vi "mac EXT ARMS TO MISS INTAKE.vi"(8 "error in (no error)":errorcluster) -> (0 "error out":errorcluster)   [LabVIEW 2020]
doc: "macro to climb from the ground to the MID bar"
uses:
  ctrl ARM MACRO ENTRY.ctl
  Robot Global Data.vi
panel:
  out "dist to extend above clearance (in)":dbl[](array[numeric])=[17.112499999999997, 13.487499999999997]
  out "clearance ht req'd (in AG)":dbl=62.125
  out "HANGAR BARS":T1={"LOW BAR AG"=48.75, "MID BAR AG"=60.25, "HIGH BAR AG"=75.625, "TRAV BAR AG"=91.0, "BAR OD"=1.66, "SPACING"=24.0}
  out "ARM Climber range":T2={"MIN"=0.0, "MAX"=22.5, "convert climber inches to tics"=18192.520379, "INITIALIZE"=-0.0625} {"convert climber inches to tics" format="%.6g"}
  out "ARM angle range":T3={"MIN"=-3.5, "MAX"=4.5, "convert arm inches to revs"=42.857, "convert arm inches to degrees"=4.96493} {"convert arm inches to degrees" format="%.6g"; "convert arm inches to revs" format="%.6g"}
  out "ARM DIMS":T4={"HOOK CTR LENGTH LEFT"=38.1375, "HOOK CTR LENGTH RIGHT"=41.7625, "HOOK DEPTH"=2.0, "HOOK ID"=1.875, "SHOULDER PIN AG"=6.875, "ARM DIFF RT-LEFT"=3.625}
  in  "Array":T6(array[cluster])=[{"LEFT"={"Climber"={"skip?"=FALSE, "CLIMBER STROKE (in)"=2.0, " speed"=0.75}, "Angle"={"skip?"=TRUE, "ARM ANGLE (deg)"=0.0, " speed"=1.0}, "DELAY (ms)"=0}, "RIGHT"={"Climber"={"skip?"=FALSE, "CLIMBER STROKE (in)"=2.0, " speed"=0.75}, "Angle"={"skip?"=TRUE, "ARM ANGLE (deg)"=0.0, " speed"=1.0}, "DELAY (ms)"=0}, "comment"={"movement"="RAISE 2.0 INCHES", "descr"=""}}] {"RIGHT"."Angle"."speed" min=0.0 max=1.0 format="%_3g"; "RIGHT"."Angle"."ARM ANGLE (deg)" format="%.3g"; "RIGHT"."Climber"."CLIMBER STROKE (in)" format="%_5g"; "RIGHT"."Climber"."speed" min=0.0 max=1.0 format="%_3g"; "LEFT"."Angle"."speed" min=0.0 max=1.0 format="%_3g"; "LEFT"."Angle"."ARM ANGLE (deg)" format="%.3g"; "LEFT"."Climber"."CLIMBER STROKE (in)" format="%_5g"; "LEFT"."Climber"."speed" min=0.0 max=1.0 format="%_3g"}
  # "22-03-15  LOW HOOKS ID measured to be about 35.5\" above shoulder pin\n35.5 + 6.875 = 42.375\" AG\n48.75\" bar - 42.375\" top ID + 2\"D + 1\" clear = 9.375\""
  # "mac EXT ARMS for MID\nExtend & angle arms to climb the MID bar\n\n1) extend arms enough to clear MID bar and angle forward\n2) angle arms rearward\n3) retract arms 4\" to grab bar\n4) retract arms and angle back to 0; leave 0.375\" buffer on right arm\n\nDO NOT FORGET TO \"MAKE CURRENT VALUES DEFAULT\""
  # "22-03-14 measured arm lengths:\nat 0% stroke, the inside hook openings were\nLEFT = 40.375\"  and RIGHT = 44.0\"\nwrt top of the shoulder arm plate"
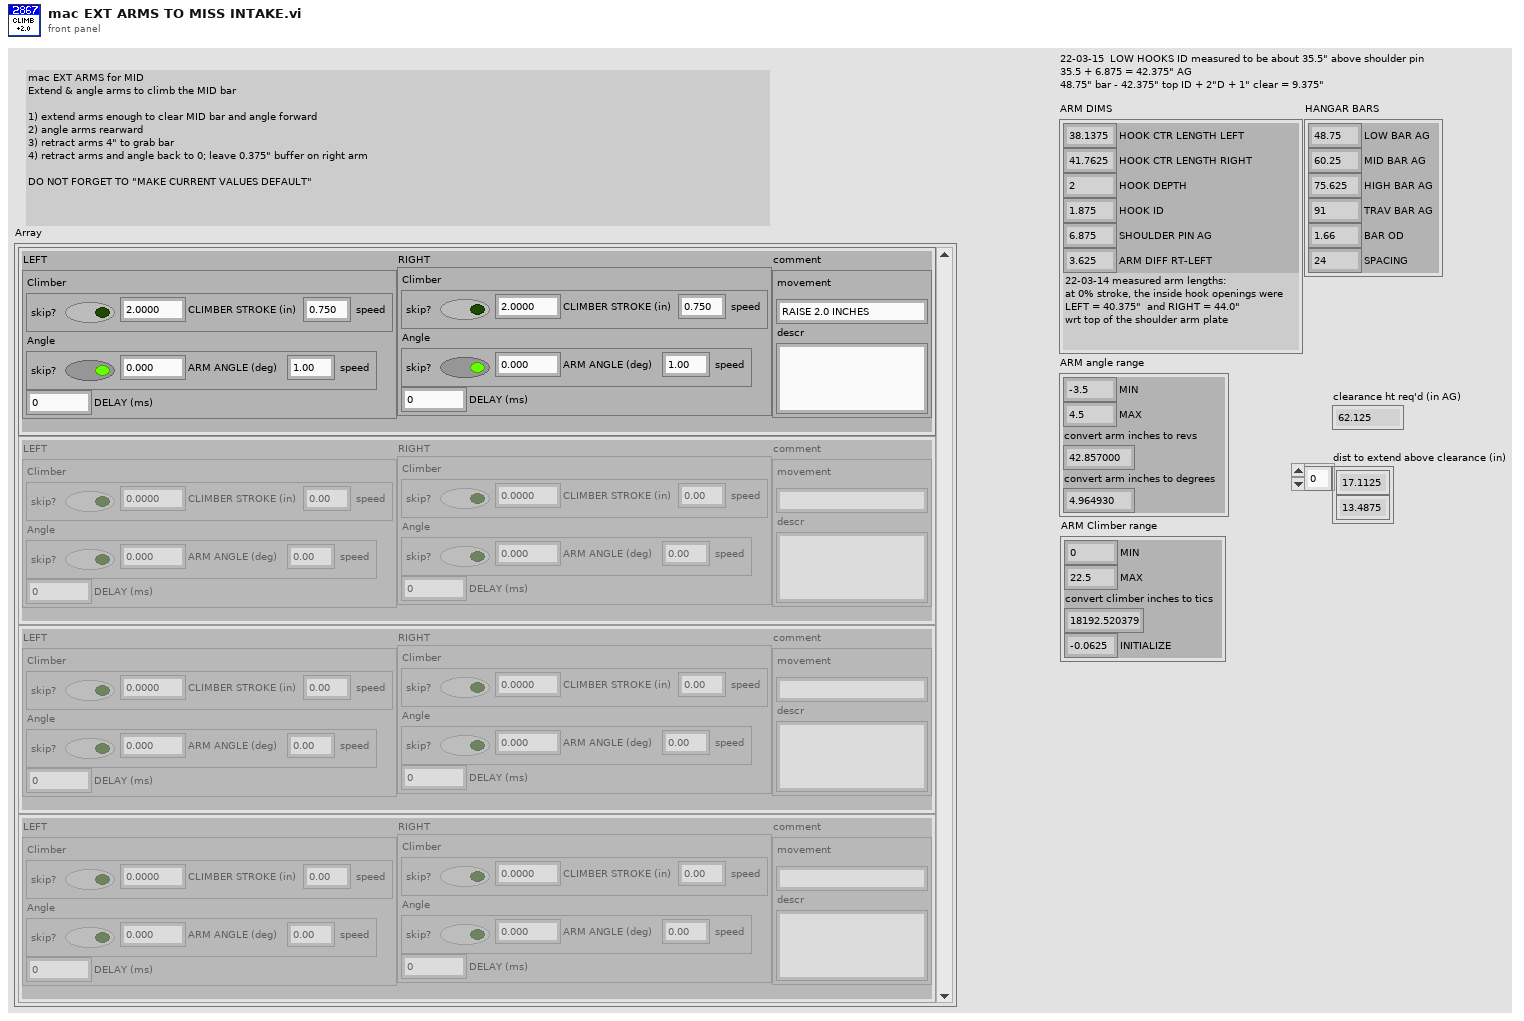
[diagram p1: front panel]
types:
  T1 = cluster{"LOW BAR AG":dbl, "MID BAR AG":dbl, "HIGH BAR AG":dbl, "TRAV BAR AG":dbl, "BAR OD":dbl, "SPACING":dbl}
  T2 = cluster{"MIN":dbl, "MAX":dbl, "convert climber inches to tics":dbl, "INITIALIZE":dbl}
  T3 = cluster{"MIN":dbl, "MAX":dbl, "convert arm inches to revs":dbl, "convert arm inches to degrees":dbl}
  T4 = cluster{"HOOK CTR LENGTH LEFT":dbl, "HOOK CTR LENGTH RIGHT":dbl, "HOOK DEPTH":dbl, "HOOK ID":dbl, "SHOULDER PIN AG":dbl, "ARM DIFF RT-LEFT":dbl}
  T5 = typedef "ctrl ARM MACRO ENTRY.ctl" = cluster{"Climber":cluster{"skip?":bool, "CLIMBER STROKE (in)":dbl, " speed":dbl}, "Angle":cluster{"skip?":bool, "ARM ANGLE (deg)":dbl, " speed":dbl}, "DELAY (ms)":u32}
  T6 = cluster{"LEFT":T5, "RIGHT":T5, "comment":cluster{"movement":string, "descr":string}}[]
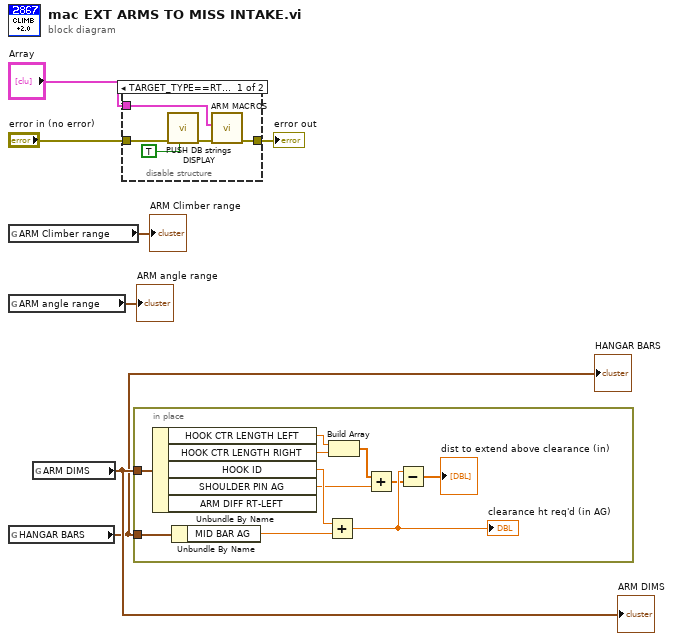
[diagram p0: block diagram]
diagram:
  n1 = global read "Robot Global Data.vi" "ARM Climber range"() -> (→"ARM Climber range":T2)
  n2 = global read "Robot Global Data.vi" "ARM angle range"() -> (→"ARM angle range":T3)
  n3 = global read "Robot Global Data.vi" "HANGAR BARS"() -> (w1:T1)
  "HANGAR BARS" <- w1
  n4 = global read "Robot Global Data.vi" "ARM DIMS"() -> (w2:T4)
  "ARM DIMS" <- w2
  n5 = disable-structure shown="TARGET_TYPE==RT, Default" {
    disable-tunnel: "Array" -> [w12 _]
    disable-tunnel: "error in (no error)" -> [w8 w13]
    disable-tunnel: [w11 w13] -> w5
    frame condition #0 (active) {
      n6 = call "PUSH DB strings DISPLAY.vi"("CLEAR LIST?"=TRUE, "error in (no error)"=w8) -> ("error out"=w9:errorcluster)  [unwired: 9 in]
      n7 = call "ARM MACROS.vi"("error in (no error)"=w9, "Array"=w12) -> ("error out"=w11:errorcluster)  [unwired: 9 in]
    }
    frame condition #1 {
    }
  }
  "error out" <- w5
  n8 = in-place {
    in-place-border: w2 -> [w24]
    in-place-border: w1 -> [w23]
    n9 = Unbundle By Name(w24) -> ("HOOK CTR LENGTH LEFT"=w20:dbl, "HOOK CTR LENGTH RIGHT"=w19:dbl, "HOOK ID"=w21:dbl, "SHOULDER PIN AG"=w17:dbl)  [unwired: 1 out]
    n10 = Unbundle By Name(w23) -> ("MID BAR AG"=w22:dbl)
    n11 = Add(x=w21, y=w22) -> (x+y=w16:dbl)
    "clearance ht req'd (in AG)" <- w16
    n12 = Build Array(w20, w19) -> (w18:dbl[])
    n13 = Add(x=w18, y=w17) -> (x+y=w15:dbl[])
    n14 = Subtract(x=w16, y=w15) -> (x-y=→"dist to extend above clearance (in)":dbl[])
  }
